vi "Pre Launch Init.vi"(11 "Panel Object Actions UI in":refnum<class "Panel Object Actions UI.lvclass">) -> (0 "error out":errorcluster, 3 "Panel Object Actions UI out":refnum<class "Panel Object Actions UI.lvclass">)   [LabVIEW 2017, in "Panel Object Actions UI.lvlib" / "Panel Object Actions UI.lvclass"]
doc: "Initializes the panel actor. Creates the Panel Helper.\n\n----\nPlease see the following web address for additional documentation and tutorial information:\nhttp://www.mooregoodideas.com/mgi-panel-manager/\n\nAuthor: Derek Trepanier\n\nCopyright (c) 2018, Moore Good Ideas, Inc.\n\nAll rights reserved.\n\nRedistribution and use in source and binary forms, with or without modification, are permitted provided that the following conditions are met:\n\n * Redistributions of source code must retain the above copyright notice, this list of conditions and the following disclaimer.\n * Redistributions in binary form must reproduce the above copyright notice, this list of conditions and the following disclaimer in the documentation and/or other materials provided with the distribution.\n * Neither the name of Moore Good Ideas, Inc. nor the names of its contributors may be used to endorse or promote products derived from this software without specific prior written permission.\n\nTHIS SOFTWARE IS PROVIDED BY THE COPYRIGHT HOLDERS AND CONTRIBUTORS \"AS IS\" AND ANY EXPRESS OR IMPLIED WARRANTIES, INCLUDING, BUT NOT LIMITED TO, THE IMPLIED WARRANTIES OF MERCHANTABILITY AND FITNESS FOR A PARTICULAR PURPOSE ARE DISCLAIMED. IN NO EVENT SHALL THE COPYRIGHT OWNER OR CONTRIBUTORS BE LIABLE FOR ANY DIRECT, INDIRECT, INCIDENTAL, SPECIAL, EXEMPLARY, OR CONSEQUENTIAL DAMAGES (INCLUDING, BUT NOT LIMITED TO, PROCUREMENT OF SUBSTITUTE GOODS OR SERVICES; LOSS OF USE, DATA, OR PROFITS; OR BUSINESS INTERRUPTION) HOWEVER CAUSED AND ON ANY THEORY OF LIABILITY, WHETHER IN CONTRACT, STRICT LIABILITY, OR TORT (INCLUDING NEGLIGENCE OR OTHERWISE) ARISING IN ANY WAY OUT OF THE USE OF THIS SOFTWARE, EVEN IF ADVISED OF THE POSSIBILITY OF SUCH DAMAGE."
uses:
  Panel Object Actions UI.lvclass
  Panel Object/Panel Object.lvclass
  Panel Object Actions UI.lvclass/Panel Object Actions UI.ctl
  <vilib>/MNProjects/Panel Manager/panel-actors/Source/Panel Actor/Panel Actor.lvclass
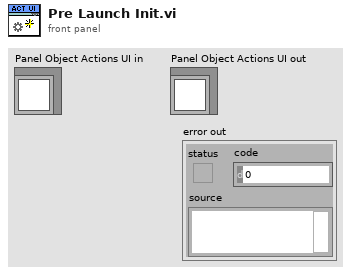
[diagram p1: front panel]
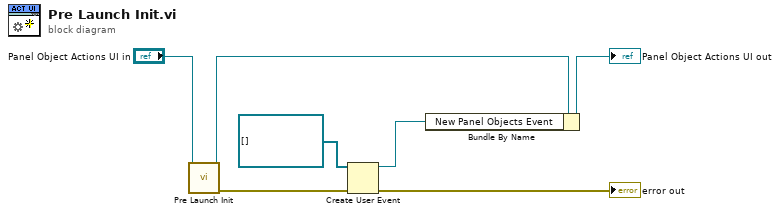
[diagram p0: block diagram]
diagram:
  n1 = call-parent "Pre Launch Init.vi"("Panel Actor in"="Panel Object Actions UI in") -> ("error out"=w7:errorcluster, "Panel Actor out"=w3:refnum<class "Panel Object Actions UI.lvclass">)  [unwired: 9 in]
  n2 = Create User Event(user event datatype=refnum<class "Panel Object.lvclass">[] [] ("Panel Objects"), error in=w7) -> (user event=w1:refnum<user-event>, error out=→"error out":errorcluster)
  n3 = Bundle By Name(cluster=w3, "New Panel Objects Event"=w1) -> (→"Panel Object Actions UI out":refnum<class "Panel Object Actions UI.lvclass">)
